vi "updateGraphs.vi"(8 "error in (no error)":errorcluster, 10 "Array":dbl[](array[numeric]), 11 "AnalysisResultsViewer in":refnum<class "AnalysisResultsViewer.lvclass">) -> (0 "error out":errorcluster, 3 "AnalysisResultsViewer out":refnum<class "AnalysisResultsViewer.lvclass">)   [LabVIEW 2011, in "Views.lvlib" / "Camera.lvlib" / "AnalysisResultsViewer.lvclass"]
uses:
  AnalysisResultsViewer.lvclass
  AnalysisResultsViewer.lvclass/AnalysisResultsViewer.ctl
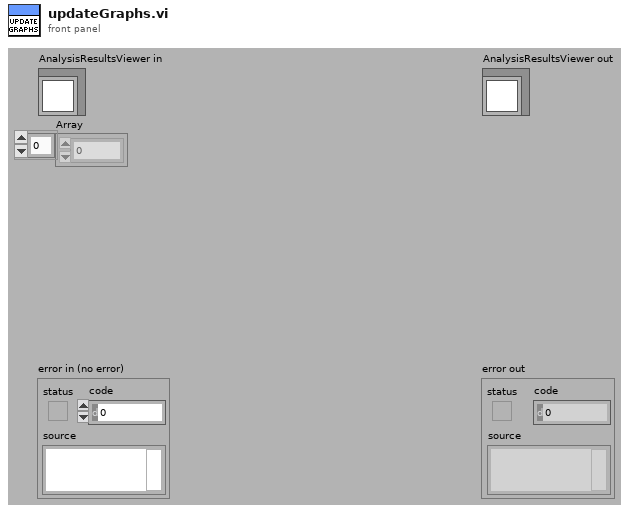
[diagram p1: front panel]
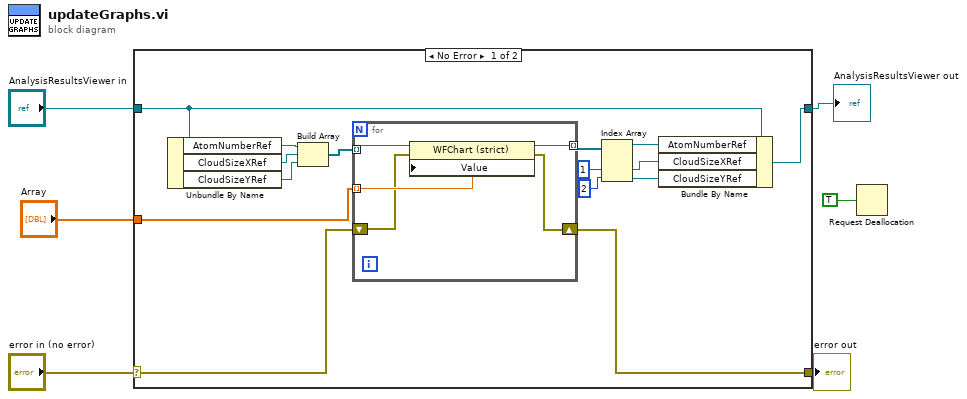
[diagram p0: block diagram]
diagram:
  n1 = case shown="No Error" "error in (no error)" {
    selector: "error in (no error)" -> [w10 w28]
    tunnel: [w9 w28] -> w5
    tunnel: [w7 w27] -> w3
    tunnel: "AnalysisResultsViewer in" -> [w8 w27]
    tunnel: "Array" -> [w11 _]
    frame No Error {
      n2 = Unbundle By Name(w8) -> ("AtomNumberRef"=w14:refnum<vi>, "CloudSizeXRef"=w13:refnum<vi>, "CloudSizeYRef"=w12:refnum<vi>)
      n3 = Build Array(w14, w13, w12) -> (w21:refnum<vi>[])
      n4 = for {
        tunnel: w21 -> [w26] mode=indexing
        tunnel: w11 -> [w25] mode=indexing
        tunnel: [w22] -> w20 mode=indexing
        shift-right: [w23] -> w9
        shift-left: w10 -> [w24]
        n5 = property class="WFChart (strict)"(reference=w26, error in=w24, "Value"=w25) -> (reference out=w22:refnum<vi>, error out=w23:errorcluster)
      }
      n6 = Index Array(array=w20, index #2=1, index #3=2) -> (element #1=w19:refnum<vi>, element #2=w17:refnum<vi>, element #3=w18:refnum<vi>)  [unwired: 1 in]
      n7 = Bundle By Name(cluster=w8, "AtomNumberRef"=w19, "CloudSizeXRef"=w17, "CloudSizeYRef"=w18) -> (w7:refnum<class "AnalysisResultsViewer.lvclass">)
    }
    frame Error {
    }
  }
  "error out" <- w5
  "AnalysisResultsViewer out" <- w3
  n8 = Request Deallocation(TRUE ("flag")) -> ()
